vi "Config Dev Field.vi"(0 "VISA resource name":refnum<visa-resource-name>, 5 "Counts (off)":enum16{"off", "on"}(ring)=enum."on", 7 "Capacitance (off)":enum16{"off", "on"}(ring)=enum."on", 9 "Loss (off)":enum16{"off", "on"}(ring)=enum."on", 11 "error in":errorcluster) -> (4 "VISA resource name out":refnum<visa-resource-name>, 15 "error out":errorcluster)   [LabVIEW 2019, in "Andeen-Hagerling 2700(400 firmware).lvlib"]
doc: "Configures which of the fields used in DMode are sent to the remote system."
uses:
  Andeen-Hagerling 2700(400 firmware).lvlib
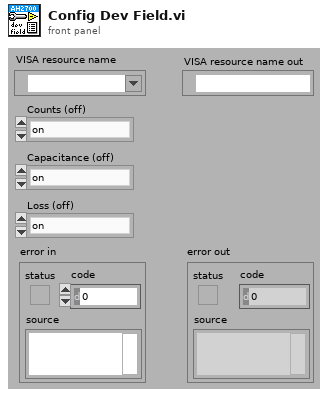
[diagram p1: front panel]
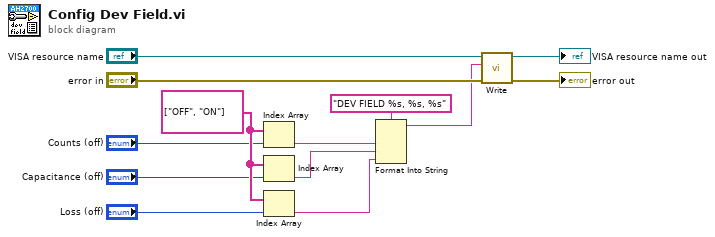
[diagram p0: block diagram]
diagram:
  w7 = string[] ["OFF", "ON"]
  n1 = Index Array(array=w7, index="Counts (off)") -> (element=w3:string)
  n2 = Index Array(array=w7, index="Capacitance (off)") -> (element=w2:string)
  n3 = Index Array(array=w7, index="Loss (off)") -> (element=w1:string)
  n4 = Format Into String(format string="DEV FIELD %s, %s, %s", w3, w2, w1) -> (resulting string=w8:string)  [unwired: 2 in, 1 out]
  n5 = call "Write.vi"("error in"="error in", "command"=w8, "VISA resource name"="VISA resource name") -> ("error out"=→"error out":errorcluster, "VISA resource name out"=→"VISA resource name out":refnum<visa-resource-name>)  [unwired: 7 in]
